vi "value to ring (CaptureMode).vi"(11 "value":string) -> (3 "CaptureMode":u32)   [LabVIEW 2020, in "AIM ARINC 664 Import.lvlib"]
uses:
  AIM ARINC 664 Import.lvlib
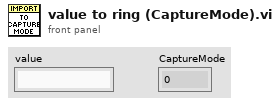
[diagram p1: front panel]
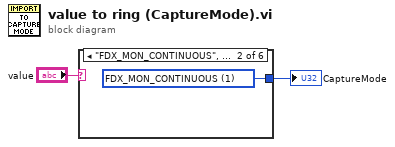
[diagram p0: block diagram]
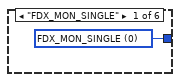
[diagram p2: hidden frame]
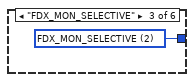
[diagram p3: hidden frame]
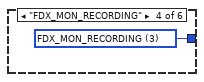
[diagram p4: hidden frame]
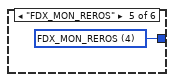
[diagram p5: hidden frame]
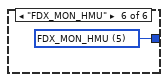
[diagram p6: hidden frame]
diagram:
  n1 = case shown="\"FDX_MON_CONTINUOUS\", Default" "value" {
    tunnel: [w3 w4 w5 w6 w7 w8] -> w2
    frame "FDX_MON_SINGLE" {
      w3 = u32 0 items=["FDX_MON_SINGLE ", "FDX_MON_CONTINUOUS", "FDX_MON_SELECTIVE", "FDX_MON_RECORDING", "FDX_MON_REROS", "FDX_MON_HMU"] ("CaptureMode")
    }
    frame "FDX_MON_CONTINUOUS", Default {
      w4 = u32 1 items=["FDX_MON_SINGLE ", "FDX_MON_CONTINUOUS", "FDX_MON_SELECTIVE", "FDX_MON_RECORDING", "FDX_MON_REROS", "FDX_MON_HMU"] ("CaptureMode")
    }
    frame "FDX_MON_SELECTIVE" {
      w5 = u32 2 items=["FDX_MON_SINGLE ", "FDX_MON_CONTINUOUS", "FDX_MON_SELECTIVE", "FDX_MON_RECORDING", "FDX_MON_REROS", "FDX_MON_HMU"] ("CaptureMode")
    }
    frame "FDX_MON_RECORDING" {
      w6 = u32 3 items=["FDX_MON_SINGLE ", "FDX_MON_CONTINUOUS", "FDX_MON_SELECTIVE", "FDX_MON_RECORDING", "FDX_MON_REROS", "FDX_MON_HMU"] ("CaptureMode")
    }
    frame "FDX_MON_REROS" {
      w7 = u32 4 items=["FDX_MON_SINGLE ", "FDX_MON_CONTINUOUS", "FDX_MON_SELECTIVE", "FDX_MON_RECORDING", "FDX_MON_REROS", "FDX_MON_HMU"] ("CaptureMode")
    }
    frame "FDX_MON_HMU" {
      w8 = u32 5 items=["FDX_MON_SINGLE ", "FDX_MON_CONTINUOUS", "FDX_MON_SELECTIVE", "FDX_MON_RECORDING", "FDX_MON_REROS", "FDX_MON_HMU"] ("CaptureMode")
    }
  }
  "CaptureMode" <- w2
